vi "Losuj pozycje startowe.vi"(8 "error in (no error)":errorcluster, 10 "Boid.lvclass":refnum<class "Boid.lvclass">, 11 "Swiat in":refnum<class "Swiat.lvclass">) -> (0 "error out":errorcluster, 3 "Swiat out":refnum<class "Swiat.lvclass">)   [LabVIEW 2014, in "Swiat.lvclass"]
uses:
  Swiat.lvclass
  Boid/Boid.lvclass
  Swiat.lvclass/Swiat.ctl
  Boid/Boid.lvclass/Boid.ctl
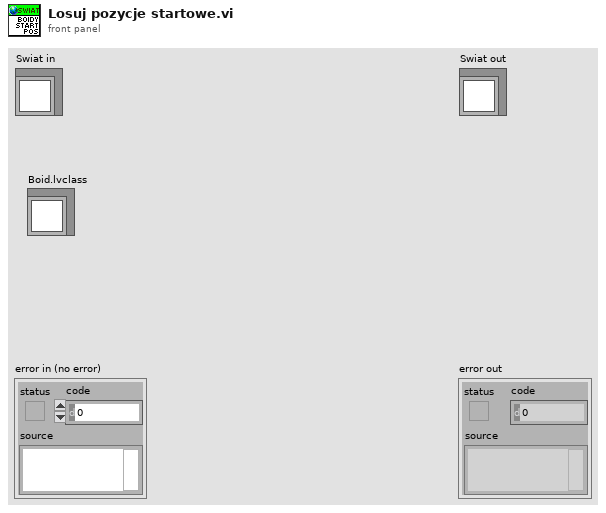
[diagram p1: front panel]
types:
  T1 = typedef "Position.ctl" = cluster{"x":i16, "y":i16}
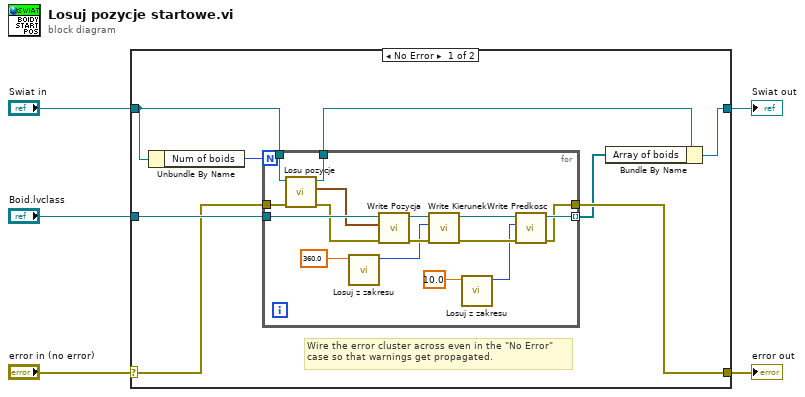
[diagram p0: block diagram]
diagram:
  n1 = case shown="No Error" "error in (no error)" {
    selector: "error in (no error)" -> [w10 w31]
    tunnel: [w9 w31] -> w4
    tunnel: [w6 w30] -> w2
    tunnel: "Swiat in" -> [w11 w30]
    tunnel: "Boid.lvclass" -> [w12 _]
    frame No Error {
      # "Wire the error cluster across even in the \"No Error\"\ncase so that warnings get propagated."
      n2 = Unbundle By Name(w11) -> ("Num of boids"=w13:i32)
      n3 = for {
        N: w13 -> [_]
        tunnel: w12 -> [w26]
        tunnel: w11 -> [w29]
        tunnel: [w28] -> w8
        tunnel: w10 -> [w27]
        tunnel: [w18] -> w9
        tunnel: [w21] -> w7 mode=indexing
        n4 = call "Losu pozycje.vi"("error in (no error)"=w27, "Swiat in"=w29) -> ("error out"=w19:errorcluster, "Random Position"=w25:T1, "Swiat out"=w28:refnum<class "Swiat.lvclass">)  [unwired: 7 in]
        n5 = call "Losuj z zakresu.vi"("Zakr"=360.0 ("y")) -> ("Wart"=w14:i16)  [unwired: 9 in, 1 out]
        n6 = call "Write Pozycja.vi"("error in (no error)"=w19, "Position"=w25, "Boid in"=w26) -> ("error out"=w23:errorcluster, "Boid out"=w24:refnum<class "Boid.lvclass">)  [unwired: 7 in]
        n7 = call "Write Kierunek.vi"("error in (no error)"=w23, "Kierunek"=w14, "Boid in"=w24) -> ("error out"=w20:errorcluster, "Boid out"=w22:refnum<class "Boid.lvclass">)  [unwired: 7 in]
        n8 = call "Losuj z zakresu.vi"("Zakr"=10.0 ("y")) -> ("Wart"=w16:i16)  [unwired: 9 in, 1 out]
        n9 = call "Write Predkosc.vi"("error in (no error)"=w20, "Predkosc"=w16, "Boid in"=w22) -> ("error out"=w18:errorcluster, "Boid out"=w21:refnum<class "Boid.lvclass">)  [unwired: 7 in]
      }
      n10 = Bundle By Name(cluster=w8, "Array of boids"=w7) -> (w6:refnum<class "Swiat.lvclass">)
    }
    frame Error {
    }
  }
  "error out" <- w4
  "Swiat out" <- w2
